vi "test-controller-acquisition.vi"() -> ()   [LabVIEW 2020]
uses:
  <vilib>/Utility/inputDevices.llb/joystickAcquire.vi
  <vilib>/Utility/inputDevices.llb/closeJoystick.vi
panel:
  out "direction info":T1
  out "axis info":T2
  out "key info":T3(array[cluster])
  out "mouse info":T4(array[cluster])
  in  "stop":bool
  out "joystick info":T5(array[cluster])
  out "button info":T6
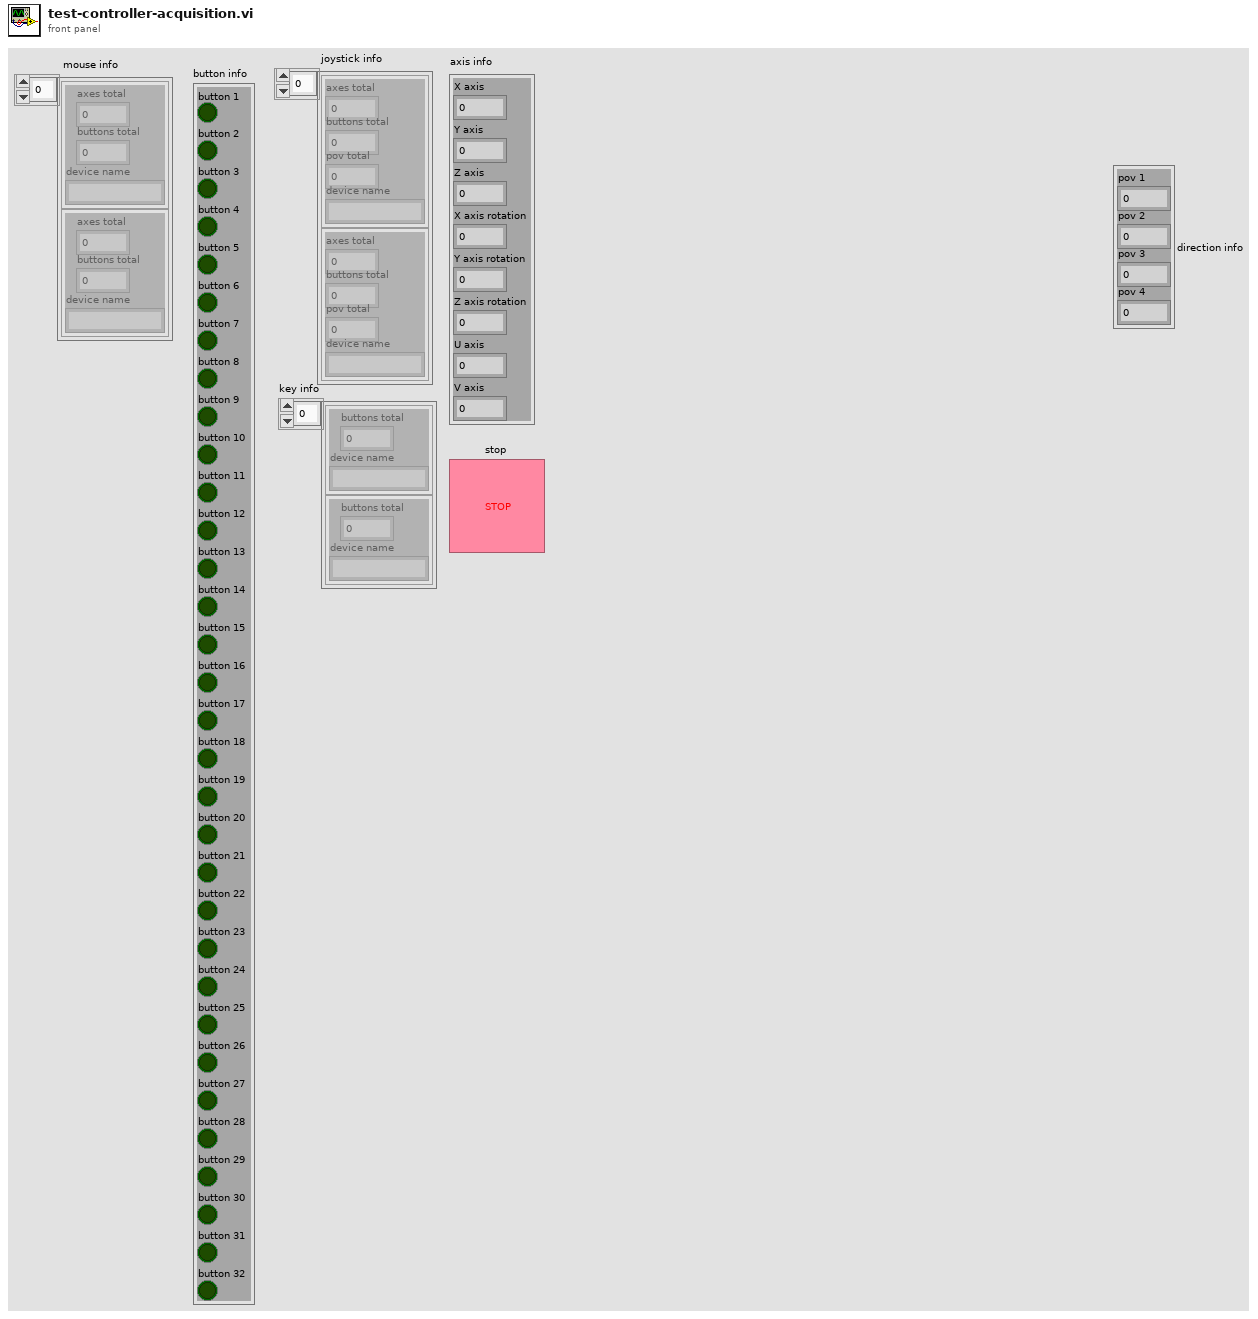
[diagram p1: front panel]
types:
  T1 = cluster{"pov 1":i32, "pov 2":i32, "pov 3":i32, "pov 4":i32}
  T2 = cluster{"X axis":i32, "Y axis":i32, "Z axis":i32, "X axis rotation":i32, "Y axis rotation":i32, "Z axis rotation":i32, "U axis":i32, "V axis":i32}
  T3 = cluster{"buttons total":u32, "device name":string}[]
  T4 = cluster{"axes total":u32, "buttons total":u32, "device name":string}[]
  T5 = cluster{"axes total":u32, "buttons total":u32, "pov total":u32, "device name":string}[]
  T6 = cluster{"button 1":bool, "button 2":bool, "button 3":bool, "button 4":bool, "button 5":bool, "button 6":bool, "button 7":bool, "button 8":bool, "button 9":bool, "button 10":bool, "button 11":bool, "button 12":bool, "button 13":bool, "button 14":bool, "button 15":bool, "button 16":bool, "button 17":bool, "button 18":bool, "button 19":bool, "button 20":bool, "button 21":bool, "button 22":bool, "button 23":bool, "button 24":bool, "button 25":bool, "button 26":bool, "button 27":bool, "button 28":bool, "button 29":bool, "button 30":bool, "button 31":bool, "button 32":bool}
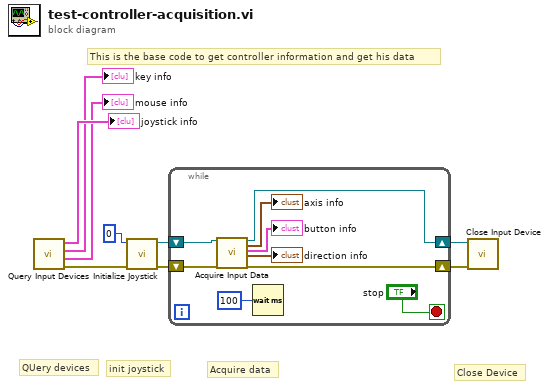
[diagram p0: block diagram]
diagram:
  # "Close Device"
  # "Acquire data"
  # "init joystick"
  # "QUery devices"
  # "This is the base code to get controller information and get his data"
  n1 = call <vilib>:"Query Input Devices.vi"() -> ("error out"=w9:errorcluster, "mouse info"=→"mouse info":T4, "key info"=→"key info":T3, "joystick info"=→"joystick info":T5)  [unwired: 8 in]
  n2 = call <vilib>:"Initialize Joystick.vi"("error in (no error)"=w9, "device index"=0) -> ("error out"=w4:errorcluster, "device ID"=w5:refnum<k1>)  [unwired: 8 in]
  n3 = while {
    shift-right: [w16] -> w3
    shift-left: w5 -> [w18]
    shift-right: [w15] -> w2
    shift-left: w4 -> [w17]
    stop <- "stop" stop-if-true
    n4 = call-poly <vilib>:"Acquire Input Data.vi"("device ID"=w18, "error in (no error)"=w17) -> ("device ID"=w16:refnum<k1>, "axis info"=→"axis info":T2, "button info"=→"button info":T6, "direction info"=→"direction info":T1, "error out"=w15:errorcluster)  [unwired: 13 in]
    n5 = Wait (ms)(milliseconds to wait=u32 100) -> ()  [unwired: 1 out]
  }
  n6 = call-poly <vilib>:"Close Input Device.vi"("error in (no error)"=w2, "device ID"=w3) -> ()  [unwired: 8 in, 1 out]
